vi "Destroy Enqueuer.vi"(8 "error in":errorcluster, 11 "QDMH in":refnum<class "QDMH.lvclass">) -> (0 "error out":errorcluster, 3 "QDMH out":refnum<class "QDMH.lvclass">)   [LabVIEW 2023, in "QDMH.lvlib" / "QDMH.lvclass"]
uses:
  QDMH.lvclass
  QDMH.lvclass/QDMH.ctl
  Custom Controls/QDMH Message.ctl
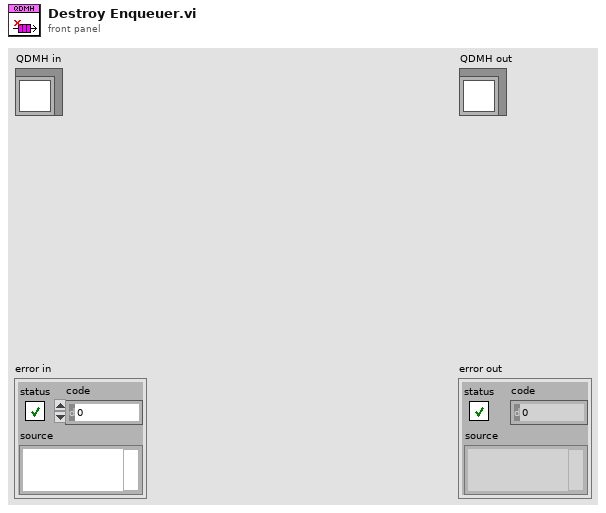
[diagram p1: front panel]
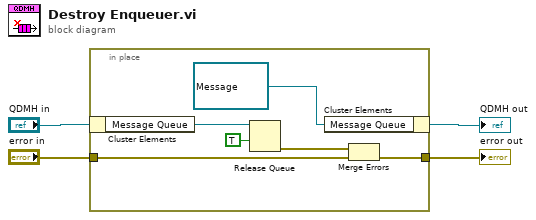
[diagram p0: block diagram]
diagram:
  n1 = in-place {
    in-place-border: [w7] -> w1
    in-place-border: "error in" -> [w5]
    n2 = in-place-cluster #1("QDMH in") -> ("Message Queue"=w10:refnum<queue>)
    n3 = Release Queue(queue=w10, force destroy? (F)=TRUE) -> (error out=w8:errorcluster)  [unwired: 1 in, 2 out]
    n4 = in-place-cluster #1("Message Queue"=refnum<queue> refnum) -> (→"QDMH out":refnum<class "QDMH.lvclass">)
    n5 = Merge Errors(w8, w5) -> (w7:errorcluster)
  }
  "error out" <- w1
